vi "All Filter string--constant.vi"() -> (3 "All Filter string":string)   [LabVIEW 2020, in "WSsupport.lvlib"]
uses:
  WSsupport.lvlib
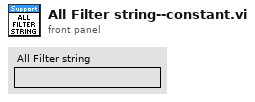
[diagram p1: front panel]
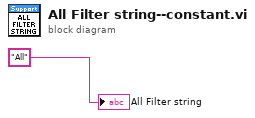
[diagram p0: block diagram]
diagram:
  "All Filter string" <- "All"
